vi "READ_MOT_ENC.vi"() -> (0 "L MOT POS":fxp<+,53,21>, 1 "R MOT POS":fxp<+,53,21>)   [LabVIEW 2019]
uses:
  <vilib>/Platform/TimedLoop/XDataNode/timing_clust.ctl
  <vilib>/Platform/TimedLoop/XDataNode/nitl_modes.ctl
  <vilib>/Platform/TimedLoop/XDataNode/wakeup.ctl
  <vilib>/rvi/Emulation/niFpgaSctlEmulationGetInTimedLoop.vi
  <vilib>/rvi/Emulation/niFpgaEmulationReportErrorSimple.vi
  <vilib>/rvi/Emulation/niFpgaGetClockAttributes.vi
  <vilib>/rvi/Emulation/niFpgaCriticalErrorInLSC.vi
  <vilib>/rvi/eio/common/nirviEmuTemplateMethod_errors.vi
  <vilib>/platform/TimedLoop/XDataNode/XDataNode.xnode
  <vilib>/eio/EIONode/EIONode.xnode
  <vilib>/Platform/TimedLoop/XDataNode/XDNodeRunTimeDep.lvlib
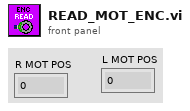
[diagram p1: front panel]
types:
  T1 = typedef "XDNodeRunTimeDep.lvlib/timing_clust.ctl" = cluster{"Expected End [f-1]":u64, "Actual End [f-1]":u64, "Finished Late? [f-1]":bool, "Expected End [i-1]":u64, "Actual End [i-1]":u64, "Finished Late? [i-1]":bool, "Expected Start [i]":u64, "Actual Start [i]":u64, "Expected Start [f]":u64, "Actual Start [f]":u64, "Source Name":string, "Structure Name":string, "Period":i64, "Deadline":i64, "Offset":i64, "Start":i64, "Priority":i32, "Timeout":i32, "Mode":T2, "Wakeup Reason":T3, "Error":errorcluster, "Source Type":string, "Secondary Source Type":string, "Global End Time":u64, "Global Start Time":u64, "Frame Duration":u64, "Iteration Duration":u64, "Assigned CPU":i32, "I/O Scan Engine Mode":u32}
  T2 = typedef "XDNodeRunTimeDep.lvlib/nitl_modes.ctl" = enum32{"No Change", "Process missed periods, maintain original phase", "Discard missed periods, maintain original phase", "Process missed periods, ignore original phase", "Discard missed periods, ignore original phase"}
  T3 = typedef "XDNodeRunTimeDep.lvlib/wakeup.ctl" = enum32{"Normal", "Aborted", "Asynchronous wakeup", "Timing source error", "Timed loop error", "Timeout"}
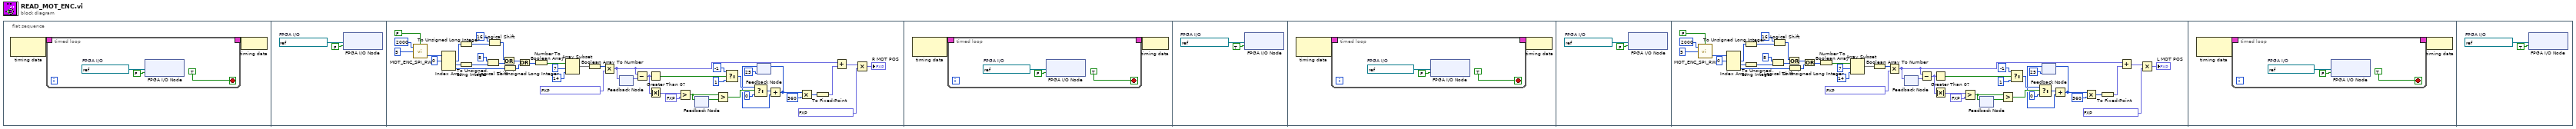
[diagram p0: block diagram]
diagram:
  n1 = flat-sequence {
    frame #0 {
      n2 = node-c288() -> (w2:T1)  [unwired: 1 in]
      n3 = timed-loop {
        timing: w2 -> [_]
        timing-out: [_] -> w1
        stop <- TRUE stop-if-true
        w4 = refnum<k21> "MOT ENC CLK"  # FPGA I/O
        n4 = xnode "FPGA I/O Node"("I/O Item"=FALSE, "FPGA I/O In"=w4) -> ()  [unwired: 1 out]
      }
      n5 = node-c288(w1) -> ()
    }
    frame #1 {
      w11 = refnum<k21> "R MOT ENC CS"  # FPGA I/O
      n6 = xnode "FPGA I/O Node"("I/O Item"=FALSE, "FPGA I/O In"=w11) -> ()  [unwired: 1 out]
    }
    frame #2 {
      n7 = call "MOT_ENC_SPI_RW.vi"("CPOL"=FALSE, "Frames to Write"=u8 5, "SPI Frequency (KHz)"=u16 2000) -> ("Data Read"=w14:u8[])  [unwired: 1 in, 1 out]
      n8 = Index Array(array=w14, index #1=0 ("index")) -> (element #1=w28:u8, element #2=w26:u8, element #3=w25:u8)  [unwired: 2 in]
      n9 = To Unsigned Long Integer(number=w28) -> (unsigned 32bit integer=w27:u32)
      n10 = To Unsigned Long Integer(number=w26) -> (unsigned 32bit integer=w22:u32)
      n11 = Logical Shift(y=i16 8, x=w22) -> (x << y=w20:u32)
      n12 = Logical Shift(y=i16 16, x=w27) -> (x << y=w16:u32)
      n13 = Or(x=w16, y=w20) -> (x .or. y?=w18:u32)
      n14 = To Unsigned Long Integer(number=w25) -> (unsigned 32bit integer=w19:u32)
      n15 = Or(x=w18, y=w19) -> (x .or. y?=w17:u32)
      n16 = Number To Boolean Array(number=w17) -> (Boolean array=w24:bool[])
      n17 = Array Subset(array=w24, index=7, length=14) -> (w12:bool[])
      n18 = Boolean Array To Number(Boolean array=w12) -> (number=w41:u16)
      n19 = Multiply(x=w41, y=fxp<+,15,-5> 0.02196979522705078) -> (x*y=w39:fxp<+,31,11>)
      n20 = feedback #1() -> (w55:fxp<+,31,11>)  [unwired: 1 in]
      n21 = feedback-in #1(w39) -> ()
      n22 = Subtract(x=w39, y=w55) -> (x-y=w53:fxp<+/-,32,12>)
      n23 = Greater Than 0?(x=w53) -> (x > 0?=w52:bool)
      n24 = Absolute Value(x=w53) -> (abs(x)=w54:fxp<+,31,11>)
      n25 = Greater?(x=w54, y=fxp<+,31,11> 180.0) -> (0:w48:bool)
      n26 = feedback #2() -> (w49:bool)  [unwired: 1 in]
      n27 = feedback-in #2(w48) -> ()
      n28 = Greater?(x=w48, y=w49) -> (0:w47:bool)
      n29 = Select(t=i16 -1, s=w52, f=i16 1) -> (s? t:f=w51:i16)
      n30 = Select(t=w51, s=w47, f=i16 0) -> (s? t:f=w50:i16)
      n31 = feedback #3(i16 25) -> (w31:i16)
      n32 = Add(x=w50, y=w31) -> (x+y=w34:i16)
      n33 = feedback-in #3(w34) -> ()
      n34 = Multiply(x=w34, y=i16 360) -> (x*y=w36:i16)
      n35 = To Fixed-Point(number=w36) -> (fixed-point=w35:fxp<+/-,16,16>)  [unwired: 1 in]
      n36 = Add(x=w39, y=w35) -> (x+y=w37:fxp<+/-,37,17>)
      n37 = Multiply(x=w37, y=fxp<+,53,33> 0.020000457763671875) -> (x*y=→"R MOT POS":fxp<+/-,64,50>)
    }
    frame #3 {
      n38 = node-c288() -> (w59:T1)  [unwired: 1 in]
      n39 = timed-loop {
        timing: w59 -> [_]
        timing-out: [_] -> w58
        stop <- TRUE stop-if-true
        w61 = refnum<k21> "MOT ENC CLK"  # FPGA I/O
        n40 = xnode "FPGA I/O Node"("I/O Item"=FALSE, "FPGA I/O In"=w61) -> ()  [unwired: 1 out]
      }
      n41 = node-c288(w58) -> ()
    }
    frame #4 {
      w68 = refnum<k21> "R MOT ENC CS"  # FPGA I/O
      n42 = xnode "FPGA I/O Node"("I/O Item"=TRUE, "FPGA I/O In"=w68) -> ()  [unwired: 1 out]
    }
    frame #5 {
      n43 = node-c288() -> (w70:T1)  [unwired: 1 in]
      n44 = timed-loop {
        timing: w70 -> [_]
        timing-out: [_] -> w69
        stop <- TRUE stop-if-true
        w72 = refnum<k21> "MOT ENC CLK"  # FPGA I/O
        n45 = xnode "FPGA I/O Node"("I/O Item"=FALSE, "FPGA I/O In"=w72) -> ()  [unwired: 1 out]
      }
      n46 = node-c288(w69) -> ()
    }
    frame #6 {
      w79 = refnum<k21> "L MOT ENC CS"  # FPGA I/O
      n47 = xnode "FPGA I/O Node"("I/O Item"=FALSE, "FPGA I/O In"=w79) -> ()  [unwired: 1 out]
    }
    frame #7 {
      n48 = call "MOT_ENC_SPI_RW.vi"("CPOL"=FALSE, "Frames to Write"=u8 5, "SPI Frequency (KHz)"=u16 2000) -> ("Data Read"=w81:u8[])  [unwired: 1 in, 1 out]
      n49 = Index Array(array=w81, index #1=0 ("index")) -> (element #1=w95:u8, element #2=w93:u8, element #3=w92:u8)  [unwired: 2 in]
      n50 = To Unsigned Long Integer(number=w95) -> (unsigned 32bit integer=w94:u32)
      n51 = To Unsigned Long Integer(number=w93) -> (unsigned 32bit integer=w89:u32)
      n52 = Logical Shift(y=i16 8, x=w89) -> (x << y=w87:u32)
      n53 = Logical Shift(y=i16 16, x=w94) -> (x << y=w83:u32)
      n54 = Or(x=w83, y=w87) -> (x .or. y?=w85:u32)
      n55 = To Unsigned Long Integer(number=w92) -> (unsigned 32bit integer=w86:u32)
      n56 = Or(x=w85, y=w86) -> (x .or. y?=w84:u32)
      n57 = Number To Boolean Array(number=w84) -> (Boolean array=w91:bool[])
      n58 = Array Subset(array=w91, index=7, length=14) -> (w80:bool[])
      n59 = Boolean Array To Number(Boolean array=w80) -> (number=w107:u16)
      n60 = Multiply(x=w107, y=fxp<+,15,-5> 0.02196979522705078) -> (x*y=w105:fxp<+,31,11>)
      n61 = feedback #4() -> (w123:fxp<+,31,11>)  [unwired: 1 in]
      n62 = feedback-in #4(w105) -> ()
      n63 = Subtract(x=w105, y=w123) -> (x-y=w121:fxp<+/-,32,12>)
      n64 = Greater Than 0?(x=w121) -> (x > 0?=w120:bool)
      n65 = Absolute Value(x=w121) -> (abs(x)=w122:fxp<+,31,11>)
      n66 = Greater?(x=w122, y=fxp<+,31,11> 180.0) -> (0:w116:bool)
      n67 = feedback #5() -> (w117:bool)  [unwired: 1 in]
      n68 = feedback-in #5(w116) -> ()
      n69 = Greater?(x=w116, y=w117) -> (0:w115:bool)
      n70 = Select(t=i16 -1, s=w120, f=i16 1) -> (s? t:f=w119:i16)
      n71 = Select(t=w119, s=w115, f=i16 0) -> (s? t:f=w118:i16)
      n72 = feedback #6(i16 25) -> (w110:i16)
      n73 = Add(x=w118, y=w110) -> (x+y=w98:i16)
      n74 = feedback-in #6(w98) -> ()
      n75 = Multiply(x=w98, y=i16 360) -> (x*y=w100:i16)
      n76 = To Fixed-Point(number=w100) -> (fixed-point=w99:fxp<+/-,16,16>)  [unwired: 1 in]
      n77 = Add(x=w105, y=w99) -> (x+y=w103:fxp<+/-,37,17>)
      n78 = Multiply(x=w103, y=fxp<+/-,53,33> 0.020000457763671875) -> (x*y=→"L MOT POS":fxp<+/-,64,48>)
    }
    frame #8 {
      n79 = node-c288() -> (w127:T1)  [unwired: 1 in]
      n80 = timed-loop {
        timing: w127 -> [_]
        timing-out: [_] -> w126
        stop <- TRUE stop-if-true
        w129 = refnum<k21> "MOT ENC CLK"  # FPGA I/O
        n81 = xnode "FPGA I/O Node"("I/O Item"=FALSE, "FPGA I/O In"=w129) -> ()  [unwired: 1 out]
      }
      n82 = node-c288(w126) -> ()
    }
    frame #9 {
      w136 = refnum<k21> "L MOT ENC CS"  # FPGA I/O
      n83 = xnode "FPGA I/O Node"("I/O Item"=TRUE, "FPGA I/O In"=w136) -> ()  [unwired: 1 out]
    }
  }
